vi "String Covert into ASCII value with binary value.vi"() -> ()   [LabVIEW 2015]
panel:
  in  "Tab Control":enum32{"Page 1", "Page 2"}(tab)
  in  "String":string
  out "unsigned byte array":u8[](array[numeric])
  out "unsigned byte array 2":u8[](array[numeric]) format="%b"
  # "String Covert into ASCII value"
  # "ASCII"
  # "Binary"
  # "Pardeep Kumar"
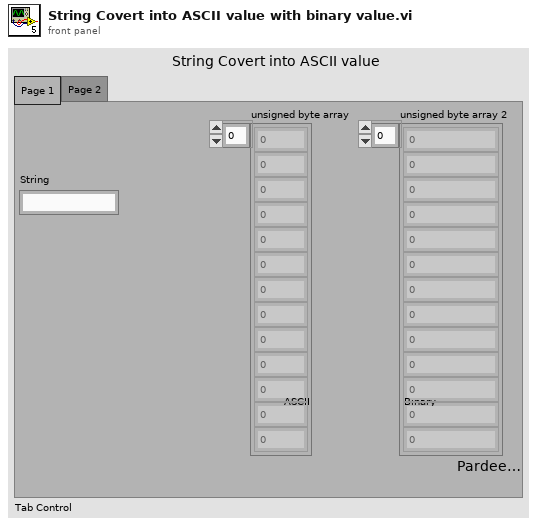
[diagram p1: front panel]
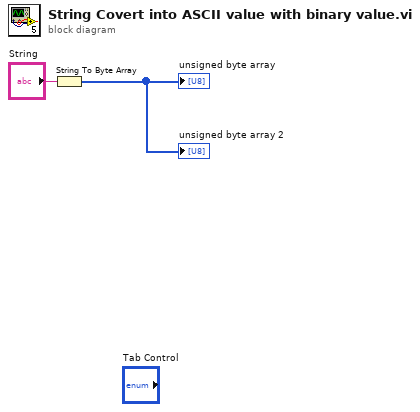
[diagram p0: block diagram]
diagram:
  n1 = String To Byte Array(string="String") -> (unsigned byte array=→"unsigned byte array" →"unsigned byte array 2":u8[])
